vi "T_step_JT.vi"   [LabVIEW 2016]
uses:
  Global/Global Variables/global.vi
  Instrument_Setup.vi
  Global/Global Variables/Data_Display_global.vi
types:
  T1 = typedef "PSIO.ctl" = cluster{"Address":T2, "Version":enum16{"PS", "IPS"}}
  T2 = typedef "OxfordAddress.ctl" = cluster{"Com Port":i32, "ISOBUS Address":i32, "GPIB Address":i16, "Communication":enum16{"RS232", "ISOBUS", "GPIB", "Gateway"}}
  T3 = typedef "LS370_Status.ctl" = cluster{"Setpoint":dbl, "MC Heater Output":dbl, "Still Heater Output":dbl, "Sorb  Heater Output":dbl, "LS370 T1":dbl, "LS370 T2":dbl, "LS370 T3":dbl, "LS370 T4":dbl, "LS370 T5":dbl, "LS370 R1":dbl, "LS370 R2":dbl, "LS370 R3":dbl, "LS370 R4":dbl, "LS370 R5":dbl, "LS370 T6":dbl, "LS370 T7":dbl, "LS370 T8":dbl, "LS370 T9":dbl, "LS370 R6":dbl, "LS370 R7":dbl, "LS370 R8":dbl, "LS370 R9":dbl, "LS370 TC-T":dbl, "LS370 TC-R":dbl}
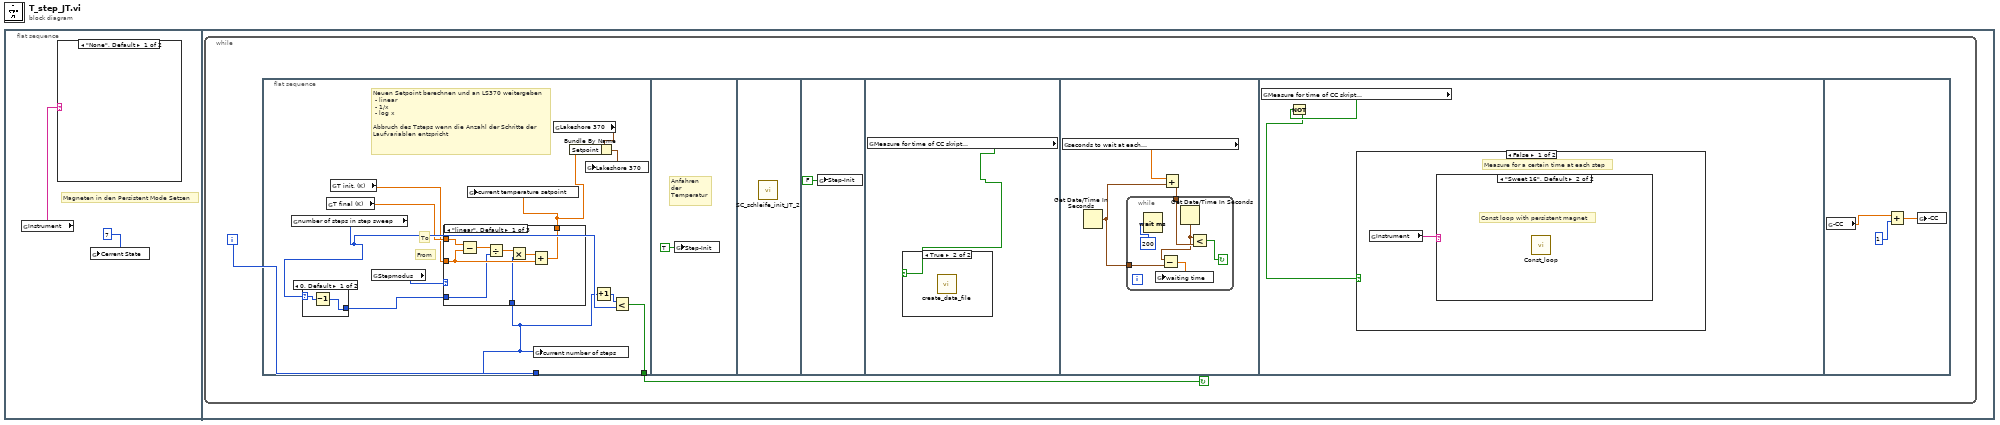
[diagram p0: block diagram]
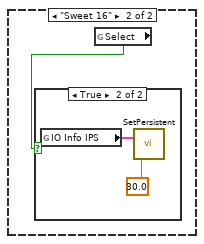
[diagram p2: hidden frame]
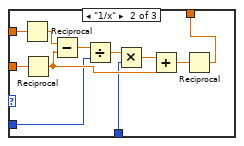
[diagram p5: hidden frame]
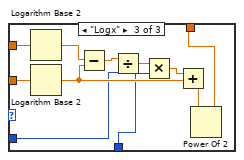
[diagram p6: hidden frame]
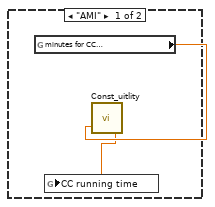
[diagram p8: hidden frame]
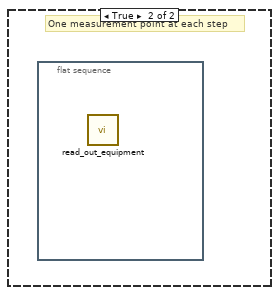
[diagram p9: hidden frame]
diagram:
  n1 = flat-sequence {
    frame #0 {
      # "Magneten in den Persistent Mode Setzen"
      n2 = global read "Instrument_Setup.vi" "Instrument"() -> (w1:string)
      n3 = case shown="\"None\", Default" w1 {
        frame "None", Default {
        }
        frame "Sweet 16" {
          n4 = global read "Data_Display_global.vi" "Select"() -> (w3:bool)
          n5 = case shown="True" w3 {
            frame False {
            }
            frame True {
              n6 = global read "Instrument_Setup.vi" "IO Info IPS"() -> (w4:T1)
              n7 = call "SetPersistent.vi"("Switch Heater Dwell Time"=dbl[unit] 30.0, "IO Info"=w4) -> ()  [unwired: 1 in, 1 out]
            }
          }
        }
      }
      n8 = global write "global.vi" "Cerrent State"(7) -> ()
    }
    frame #1 {
      n9 = while {
        i -> [w7]
        stop <- w6 continue-if-true
        n10 = flat-sequence {
          tunnel: w7 -> [w11]
          tunnel: [w12] -> w6
          frame #0 {
            # "Neuen Setpoint berechnen und an LS370 weitergeben\n - linear\n - 1/x\n - log x\n\nAbbruch des Tsteps wenn die Anzahl der Schritte der \nLaufvariablen entspricht"
            # "From"
            # "To"
            n11 = global read "global.vi" "number of steps in step sweep"() -> (w16:i32)
            n12 = case shown="0, Default" w16 {
              selector: w16 -> [w20 w21]
              tunnel: [w19 w21] -> w17
              frame 0, Default {
                n13 = Decrement(x=w20) -> (x-1=w19:i32)
              }
              frame 1 {
              }
            }
            n14 = global read "global.vi" "T final (K)"() -> (w14:dbl)
            n15 = global read "global.vi" "T init. (K)"() -> (w13:dbl)
            n16 = global read "Instrument_Setup.vi" "Stepmodus"() -> (w15:enum16{"linear", "1/x", "Logx"})
            n17 = case shown="\"linear\", Default" w15 {
              tunnel: w14 -> [w29 w39 w51]
              tunnel: w13 -> [w26 w40 w50]
              tunnel: [w24 w34 w43] -> w9
              tunnel: w17 -> [w23 w31 w42]
              tunnel: w11 -> [w22 w30 w41]
              frame "linear", Default {
                n18 = Subtract(x=w29, y=w26) -> (x-y=w28:dbl)
                n19 = Divide(x=w28, y=w23) -> (x/y=w27:dbl)
                n20 = Multiply(x=w27, y=w22) -> (x*y=w25:dbl)
                n21 = Add(x=w25, y=w26) -> (x+y=w24:dbl)
              }
              frame "1/x" {
                n22 = Reciprocal(x=w39) -> (1/x=w33:dbl)
                n23 = Reciprocal(x=w40) -> (1/x=w32:dbl)
                n24 = Subtract(x=w33, y=w32) -> (x-y=w38:dbl)
                n25 = Divide(x=w38, y=w31) -> (x/y=w37:dbl)
                n26 = Multiply(x=w37, y=w30) -> (x*y=w36:dbl)
                n27 = Add(x=w36, y=w32) -> (x+y=w35:dbl)
                n28 = Reciprocal(x=w35) -> (1/x=w34:dbl)
              }
              frame "Logx" {
                n29 = Logarithm Base 2(1:w51) -> (0:w49:dbl)
                n30 = Logarithm Base 2(1:w50) -> (0:w45:dbl)
                n31 = Subtract(x=w49, y=w45) -> (x-y=w48:dbl)
                n32 = Divide(x=w48, y=w42) -> (x/y=w47:dbl)
                n33 = Multiply(x=w47, y=w41) -> (x*y=w46:dbl)
                n34 = Add(x=w46, y=w45) -> (x+y=w44:dbl)
                n35 = Power Of 2(x=w44) -> (2^x=w43:dbl)
              }
            }
            n36 = global write "Data_Display_global.vi" "current temperature setpoint"(w9) -> ()
            n37 = global write "Data_Display_global.vi" "current number of steps"(w11) -> ()
            n38 = global read "Data_Display_global.vi" "Lakeshore 370"() -> (w10:T3)
            n39 = Bundle By Name(cluster=w10, "Setpoint"=w9) -> (w8:T3)
            n40 = global write "Data_Display_global.vi" "Lakeshore 370"(w8) -> ()
            n41 = Increment(x=w11) -> (x+1=w18:i32)
            n42 = Less?(x=w18, y=w16) -> (x < y?=w12:bool)
          }
          frame #1 {
            # "Anfahren \nder \nTemperatur"
            n43 = global write "global.vi" "Step-Init"(TRUE) -> ()
          }
          frame #2 {
            n44 = call "SC_schleife_init_JT_2.vi"() -> ()  [unwired: 4 in]
          }
          frame #3 {
            n45 = global write "global.vi" "Step-Init"(FALSE) -> ()
          }
          frame #4 {
            n46 = global read "Instrument_Setup.vi" "Measure for time of CC skript\nat each field step point"() -> (w54:bool)
            n47 = case shown="True" w54 {
              frame False {
              }
              frame True {
                n48 = call "create_data_file.vi"() -> ()  [unwired: 3 in]
              }
            }
          }
          frame #5 {
            n49 = global read "Instrument_Setup.vi" "seconds to wait at each\nfield step in a step sweep"() -> (w55:dbl)
            n50 = Get Date/Time In Seconds() -> (seconds since 1Jan1904=w56:timestamp)
            n51 = Add(x=w55, y=w56) -> (x+y=w57:timestamp)
            n52 = while {
              tunnel: w57 -> [w63]
              tunnel: w56 -> [w59]
              stop <- w62 continue-if-true
              n53 = Wait (ms)(milliseconds to wait=u32 200) -> ()  [unwired: 1 out]
              n54 = Get Date/Time In Seconds() -> (seconds since 1Jan1904=w60:timestamp)
              n55 = Subtract(x=w60, y=w59) -> (x-y=w58:dbl)
              n56 = global write "Data_Display_global.vi" "waiting time"(w58) -> ()
              n57 = Less?(x=w60, y=w63) -> (x < y?=w62:bool)
            }
          }
          frame #6 {
            n58 = global read "Instrument_Setup.vi" "Measure for time of CC skript\nat each field step point"() -> (w65:bool)
            n59 = Not(x=w65) -> (.not. x?=w64:bool)
            n60 = case shown="False" w64 {
              frame False {
                # "Measure for a certain time at each step"
                n61 = global read "Instrument_Setup.vi" "Instrument"() -> (w66:string)
                n62 = case shown="\"Sweet 16\", Default" w66 {
                  frame "AMI" {
                    n63 = global read "Instrument_Setup.vi" "minutes for CC\nto run"() -> (w68:dbl)
                    n64 = call "Const_uitlity.vi"("Duration"=w68) -> ("Minutes passed"=w67:dbl)  [unwired: 1 in]
                    n65 = global write "Data_Display_global.vi" "CC running time"(w67) -> ()
                  }
                  frame "Sweet 16", Default {
                    # "Const loop with persistent magnet"
                    n66 = call "Const_loop.vi"() -> ()  [unwired: 4 in]
                  }
                }
              }
              frame True {
                # "One measurement point at each step"
                n67 = flat-sequence {
                  frame #0 {
                    n68 = call "read_out_equipment.vi"() -> ()  [unwired: 1 in]
                  }
                }
              }
            }
          }
          frame #7 {
            n69 = global read "global.vi" "-CC"() -> (w71:dbl)
            n70 = Add(x=w71, y=1) -> (x+y=w69:dbl)
            n71 = global write "global.vi" "-CC"(w69) -> ()
          }
        }
      }
    }
  }
